vi "Assemble QuadViewManager.vi"(8 "Bottom-Right View":refnum<class "IViewable.lvclass">, 9 "Bottom-Left View":refnum<class "IViewable.lvclass">, 10 "Top-Right View":refnum<class "IViewable.lvclass">, 11 "Top-Left View":refnum<class "IViewable.lvclass">) -> (3 "QuadViewManager out":refnum<class "QuadViewManager.lvclass">)   [LabVIEW 2020, in "QuadViewManager.lvlib" / "QuadViewManager.lvclass"]
doc: "组装四视图管理器"
uses:
  QuadViewManager.lvclass
  modules/mva-viewable/Source/IViewable/IViewable/IViewable.lvclass
  modules/mva-viewable/Source/IViewManager/IViewManager Messages/Launch Nested Views Msg/Launch Nested Views Msg.lvclass/Launch Nested Views Msg.ctl
  modules/mva-viewable/Source/IViewManager/IViewManager/IViewManager.lvclass/IViewManager.ctl
  modules/mva-viewable/Source/IViewManager/IViewManager Messages/Launch Nested Views Msg/Pack Launch Nested Views Msg.vi
  modules/mva-viewable/Source/IViewManager/IViewManager Messages/Launch Nested Views Msg/Launch Nested Views Msg.lvclass
  modules/mva-viewable/Source/IViewManager/IViewManager/IViewManager.lvclass
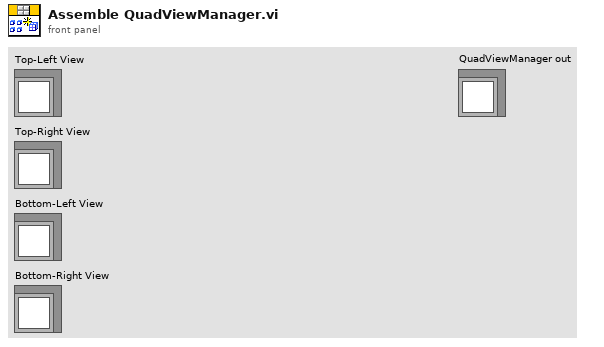
[diagram p1: front panel]
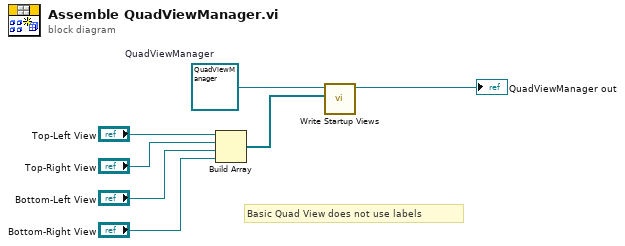
[diagram p0: block diagram]
diagram:
  w7 = refnum<class "QuadViewManager.lvclass"> refnum  # QuadViewManager
  # "Basic Quad View does not use labels"
  n1 = Build Array("Top-Left View", "Top-Right View", "Bottom-Left View", "Bottom-Right View") -> (w1:refnum<class "IViewable.lvclass">[])
  n2 = call "Write Startup Views.vi"("Startup Views"=w1, "IViewManager in"=w7) -> ("IViewManager out"=→"QuadViewManager out":refnum<class "QuadViewManager.lvclass">)  [unwired: 9 in]
